vi "J1939 Message DM13 Stop.vi"(0 "Source Address":u8=27, 7 "DA":u8) -> (4 "ID":u32 format="%.0x", 8 "Data":u8[](array[numeric]) format="%.0x")   [LabVIEW 2013, in "J1939.lvlib"]
uses:
  J1939.lvlib
  API Types/PGN Fields Cluster.ctl
  Frame Conversion/Convert J1939 ID to CAN Arb ID.vi
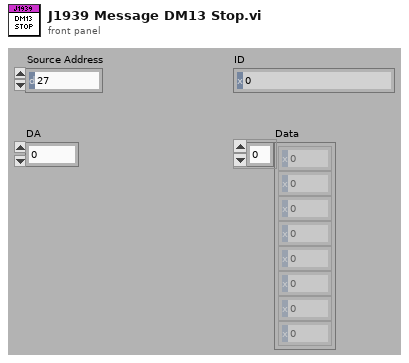
[diagram p1: front panel]
types:
  T1 = typedef "J1939.lvlib/PGN Fields Cluster.ctl" = cluster{"Reserved Bit":u8, "Data page":u8, "PDU Format":u8, "PDU Specific":u8}
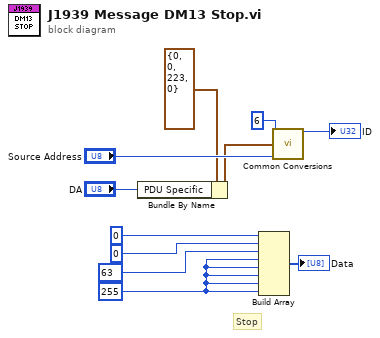
[diagram p0: block diagram]
diagram:
  w8 = u8 255
  # "Stop"
  n1 = Bundle By Name(cluster=T1 {"Reserved Bit"=0, "Data page"=0, "PDU Format"=223, "PDU Specific"=0} ("PGN Fields"), "PDU Specific"="DA") -> (w1:T1)
  n2 = Build Array(u8 0, u8 0, u8 63, w8, w8, w8, w8, w8) -> (→"Data":u8[])
  n3 = call-poly "Common Conversions.vi"("Priority"=u8 6, "PGN Fields"=w1, "Source Address"="Source Address") -> ("ID"=→"ID":u32)  [unwired: 11 in, 1 out]
